vi "NPC3SG Set Loop.vi"(2 "Get  Error":errorcluster caption="Fehler (Eingang)", 3 "Close Loop?":bool, 4 "Drive Visa Name":refnum<visa-resource-name>) -> (0 "Send Error":errorcluster caption="Fehler (Ausgang)", 1 "Success?":bool)   [LabVIEW 2010]
uses:
  drivers/Newport NPC3SG/SubNPC3SG.llb/device variables.vi
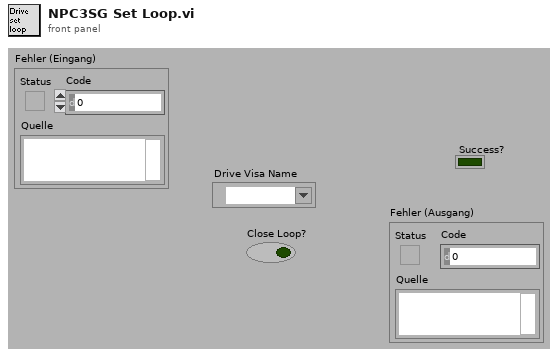
[diagram p1: front panel]
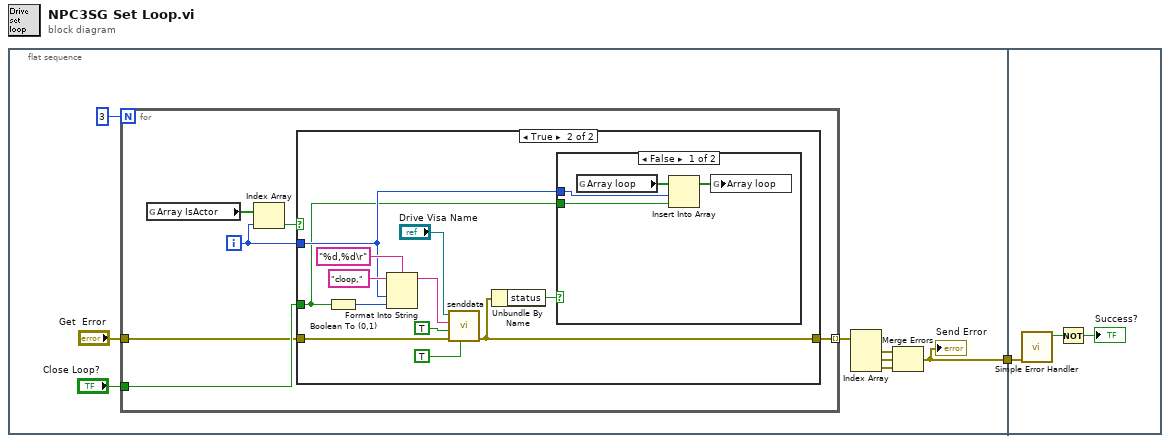
[diagram p0: block diagram]
diagram:
  n1 = flat-sequence {
    tunnel: [w2] -> w1
    tunnel: w1 -> [w33]
    frame #0 {
      n2 = for {
        N: 3 -> [_]
        tunnel: "Close Loop?" -> [w15]
        tunnel: "Get  Error" -> [w13]
        tunnel: [w14] -> w3 mode=indexing
        i -> [w10]
        n3 = global read "device variables.vi" "Array IsActor"() -> (w12:bool[])
        n4 = Index Array(array=w12, index=w10) -> (element=w11:bool)
        n5 = case shown="True" w11 {
          tunnel: w15 -> [_ w18]
          tunnel: w10 -> [_ w19]
          tunnel: [w16 w20] -> w14
          tunnel: w13 -> [w16 w22]
          frame False {
          }
          frame True {
            n6 = Boolean To (0,1)(Boolean=w18) -> (0, 1=w26:i16)
            n7 = Format Into String(format string="%d,%d\r" ("Format-String"), initial string="cloop,", w19, w26) -> (resulting string=w24:string)  [unwired: 1 in, 1 out]
            n8 = call "senddata.vi"("read ERR"=TRUE, "error in"=w22, "write Command"=TRUE, "writebuffer"=w24, "VISA-Ressourcen-Name"="Drive Visa Name") -> ("error out"=w20:errorcluster)  [unwired: 4 in, 2 out]
            n9 = Unbundle By Name(w20) -> ("status"=w21:bool)
            n10 = case shown="False" w21 {
              tunnel: w18 -> [w30 _]
              tunnel: w19 -> [w29 _]
              frame False {
                n11 = global read "device variables.vi" "Array loop"() -> (w32:bool[])
                n12 = Insert Into Array(array=w32, index=w29, new element=w30) -> (w31:bool[])
                n13 = global write "device variables.vi" "Array loop"(w31) -> ()
              }
              frame True {
              }
            }
          }
        }
      }
      n14 = Index Array(array=w3) -> (element #1=w6:errorcluster, element #2=w5:errorcluster, element #3=w4:errorcluster)  [unwired: 3 in]
      n15 = Merge Errors(w6, w5, w4) -> (w2:errorcluster)
      "Send Error" <- w2
    }
    frame #1 {
      n16 = call <vilib>:"Simple Error Handler.vi"("error in (no error)"=w33) -> ("error?"=w35:bool)  [unwired: 4 in, 4 out]
      n17 = Not(x=w35) -> (.not. x?=→"Success?":bool)
    }
  }
